vi "Untitled 2.vi"() -> ()   [LabVIEW 2021]
panel:
  in  "Listbox":i32(listbox)
  in  "Multicolumn Listbox":i32(listbox)
  out "Table":string[][](table)
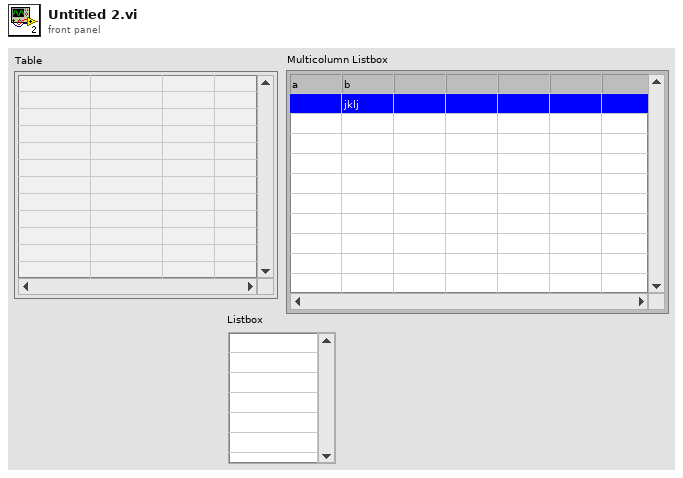
[diagram p1: front panel]
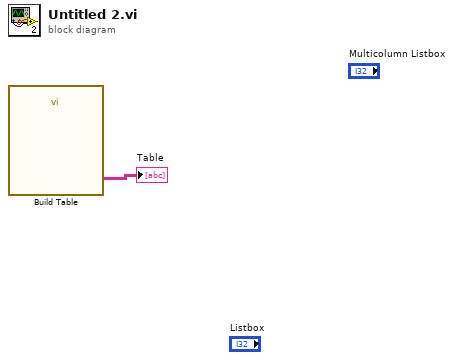
[diagram p0: block diagram]
diagram:
  n1 = call "Build Table"() -> ("Table"=→"Table":string[][])  [unwired: 5 in, 6 out]
